vi "Add_filename_suffix.vi"(0 "Filename":string, 1 "Suffix to add":string) -> (2 "Original Suffix":string, 3 "Filename out":string, 4 "Base name":string, 5 "Extension length":i32)   [LabVIEW 2018]
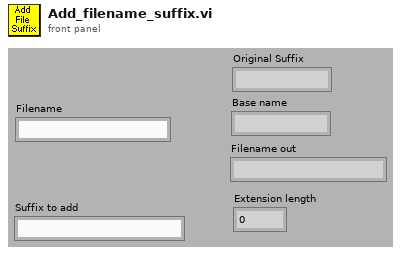
[diagram p1: front panel]
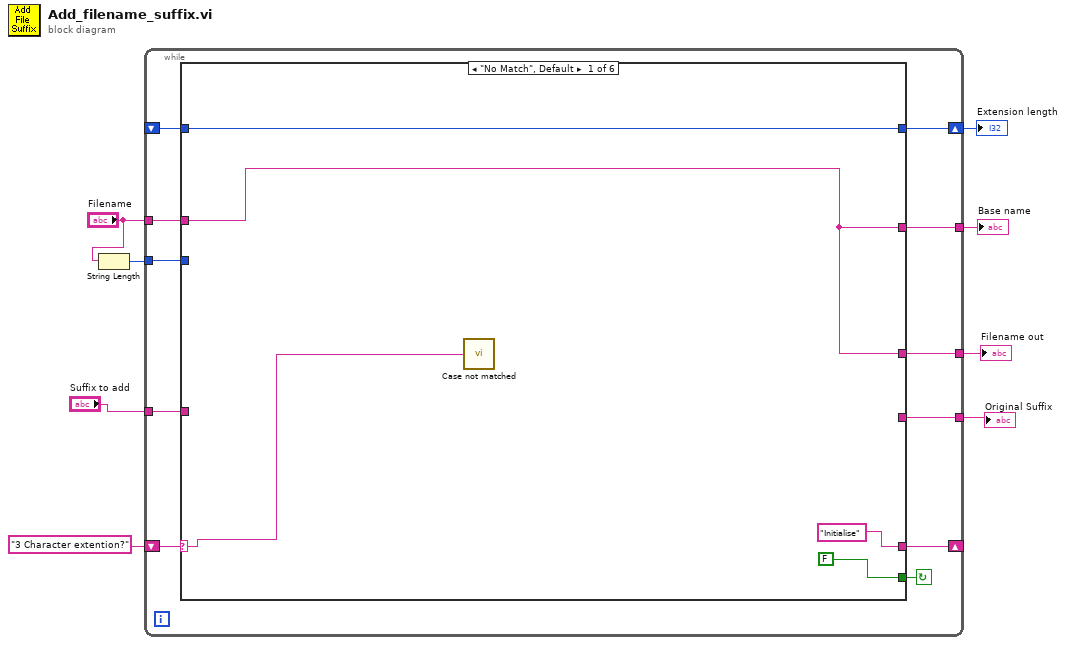
[diagram p0: block diagram]
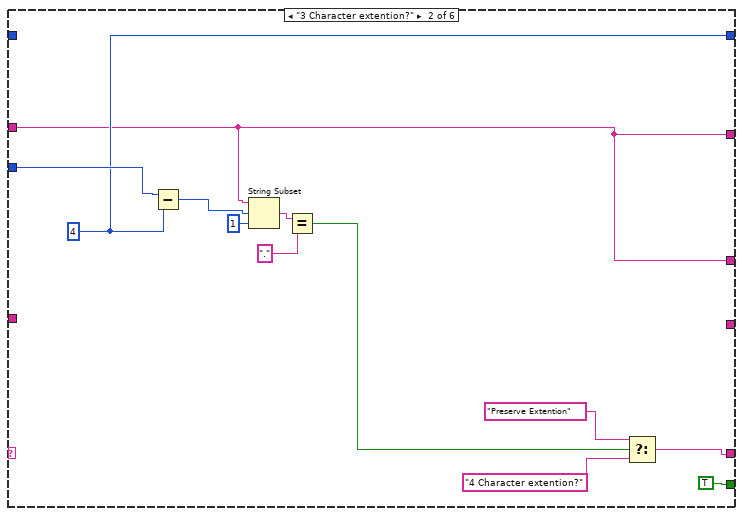
[diagram p2: hidden frame]
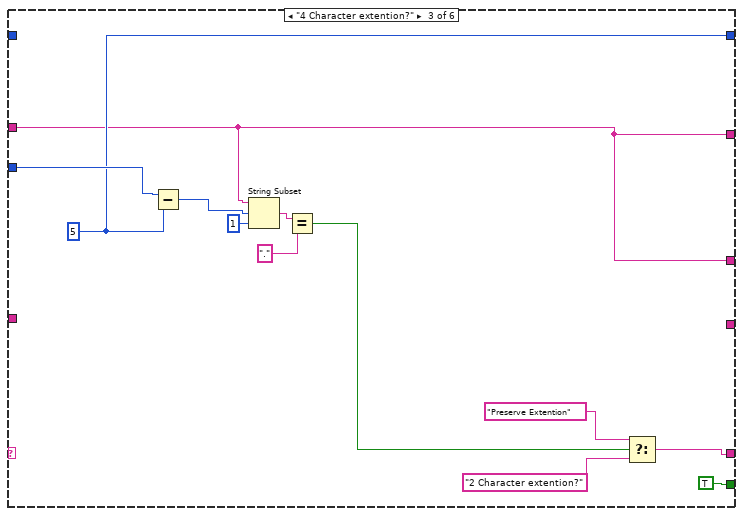
[diagram p3: hidden frame]
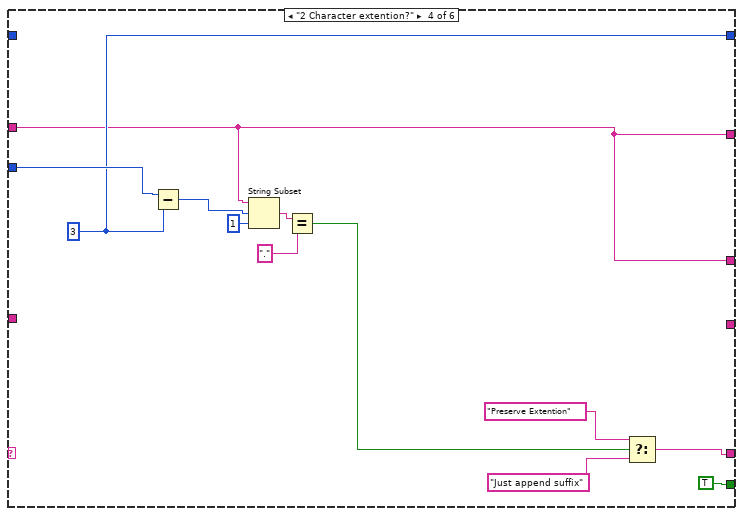
[diagram p4: hidden frame]
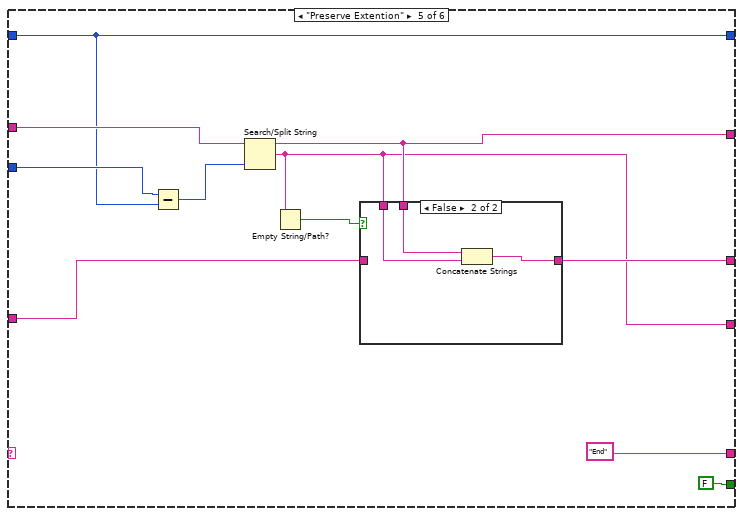
[diagram p5: hidden frame]
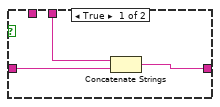
[diagram p6: hidden frame]
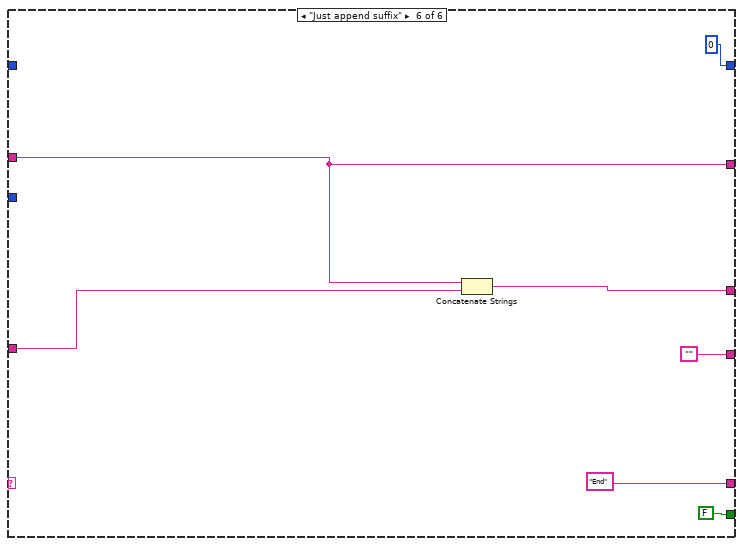
[diagram p7: hidden frame]
diagram:
  n1 = String Length(string="Filename") -> (length=w7:i32)
  n2 = while {
    shift-left: "3 Character extention?" -> [w17]
    shift-right: [w18] -> _
    tunnel: w7 -> [w16]
    tunnel: "Filename" -> [w15]
    tunnel: "Suffix to add" -> [w14]
    tunnel: [w13] -> w4
    shift-right: [w12] -> w3
    shift-left: _ -> [w11]
    tunnel: [w10] -> w2
    tunnel: [w9] -> w1
    stop <- w19 continue-if-true
    n3 = case shown="\"No Match\", Default" w17 {
      selector: w17 -> [w20 _ _ _ _ _]
      tunnel: [FALSE TRUE TRUE TRUE FALSE FALSE] -> w19
      tunnel: ["Initialise" w27 w39 w51 "End" "End"] -> w18
      tunnel: w16 -> [_ w35 w47 w59 w69 _]
      tunnel: w15 -> [w21 w25 w37 w49 w67 w79]
      tunnel: w14 -> [_ _ _ _ w63 w82]
      tunnel: [w21 w25 w37 w49 w66 w81] -> w13
      tunnel: [w22 w30 w42 w54 w65 0 ("y")] -> w12
      tunnel: w11 -> [w22 _ _ _ w65 _]
      tunnel: [w21 w25 w37 w49 w64 w79] -> w10
      tunnel: [_ _ _ _ w61 ""] -> w9
      frame "No Match", Default {
        n4 = call "Case not matched.vi"("Case Name not Matched"=w20) -> ()
      }
      frame "3 Character extention?" {
        w30 = 4 ("y")
        n5 = Subtract(x=w35, y=w30) -> (x-y=w32:i32)
        n6 = String Subset(string=w25, offset (0)=w32, length (rest)=1 ("length (rest)")) -> (substring=w31:string)
        n7 = Equal?(x=w31, y=".") -> (x = y?=w29:bool)
        n8 = Select(t="Preserve Extention", s=w29, f="4 Character extention?") -> (s? t:f=w27:string)
      }
      frame "4 Character extention?" {
        w42 = 5 ("y")
        n9 = Subtract(x=w47, y=w42) -> (x-y=w44:i32)
        n10 = String Subset(string=w37, offset (0)=w44, length (rest)=1 ("length (rest)")) -> (substring=w43:string)
        n11 = Equal?(x=w43, y=".") -> (x = y?=w41:bool)
        n12 = Select(t="Preserve Extention", s=w41, f="2 Character extention?") -> (s? t:f=w39:string)
      }
      frame "2 Character extention?" {
        w54 = 3 ("y")
        n13 = Subtract(x=w59, y=w54) -> (x-y=w56:i32)
        n14 = String Subset(string=w49, offset (0)=w56, length (rest)=1 ("length (rest)")) -> (substring=w55:string)
        n15 = Equal?(x=w55, y=".") -> (x = y?=w53:bool)
        n16 = Select(t="Preserve Extention", s=w53, f="Just append suffix") -> (s? t:f=w51:string)
      }
      frame "Preserve Extention" {
        n17 = Subtract(x=w69, y=w65) -> (x-y=w68:i32)
        n18 = Search/Split String(string=w67, offset (0)=w68) -> (substring before match=w64:string, match + rest of string=w61:string)  [unwired: 2 out]
        n19 = Empty String/Path?(string/path=w61) -> (empty?=w62:bool)
        n20 = case shown="False" w62 {
          tunnel: w61 -> [_ w77]
          tunnel: [w74 w76] -> w66
          tunnel: w64 -> [w73 w75]
          tunnel: w63 -> [w72 _]
          frame True {
            n21 = Concatenate Strings(w73, w72) -> (w74:string)
          }
          frame False {
            n22 = Concatenate Strings(w75, w77) -> (w76:string)
          }
        }
      }
      frame "Just append suffix" {
        n23 = Concatenate Strings(w79, w82) -> (w81:string)
      }
    }
  }
  "Filename out" <- w4
  "Extension length" <- w3
  "Base name" <- w2
  "Original Suffix" <- w1
